vi "Read SCH Array Parameters.vi"(7 "FPGA Configuration Values In":T1={"Ln2 Filter Size"=10, "VT Quench Tick Limit"=4000000, "VT Quench Volt Limit"=0.1999969482421875, "Joint Tick Limit"=4000000, "Joint Volt Limit"=9.98377799987793e-07, "CoWound Volt Limit"=0.20001220703125, "CoWound Tick Limit"=4000000, "SC Bus Limit"=0.001953125, "SC Bus Tick Limit"=4000000, "ResMag Tick Limit"=1000000, "DAQ Cycle Ticks"=4096, "Res Mag dI/dt Delay"=256, "dI/dT scaling"=38.14697265625, "Pressure Inlet Limit (BarA)"=6.0, "Bore Tube Volt Limit"=0.5999999940395355, "Pressure Outlet Limit (BarA)"=5.0, "Activation Current (kA)"=0.5, "Dump Resistor Scale Factor"=200.0, "Co-Wound Asymmetry Factor"=0.0, "Co-Wound Scale Factor"=200.0, "Layer Scale Factors"=[3.0, 3.0, 3.0, 3.0, 3.0, 3.0, 3.0, 3.0, 3.0, 3.0, 3.0, 3.0, 3.0, 3.0, 3.0, 3.0, 3.0, 3.0], "Fudge Factors"=[0.0, 0.0, 0.0, 0.0, 0.0, 0.0, 0.0, 0.0, 0.0, 0.0, 0.0, 0.0, 0.0, 0.0, 0.0, 0.0], "Joint Scale Factors"=[1.0013580322265625e-05, 1.0013580322265625e-05, 1.0013580322265625e-05, 1.0013580322265625e-05, 1.0013580322265625e-05, 1.0013580322265625e-05, 1.0013580322265625e-05, 1.0013580322265625e-05], "SC Bus Scale"=[0.0009765326976776123, 0.0009765326976776123, 0.0009765326976776123, 0.0009765326976776123, 0.0009765326976776123, 0.0009765326976776123], "Pressure Scale Factor"=[1.723690003156662, 1.723690003156662, 1.723690003156662, 1.723690003156662], "# Consecutive Zeros Fault"=1000, "Digitize Convert Ticks"=200, "Digitize Reset Ticks"=400, "Convert Clock Ticks"=20, "Digitize Read Delay Ticks"=13, "Digitize # Bits"=16, "HTS Lead Tick Limit"=4000000, "Res Lead Tick Limit"=4000000, "HTS Lead Trip"=0.20000000298023224, "Res Lead Limit"=0.001953125, "HTS Lead FRZ"=0.006999999284744263, "HTS Lead Warn"=0.0010000020265579224} {"HTS Lead Warn" format="%_6g"; "HTS Lead FRZ" format="%_6g"; "Res Lead Limit" format="%_6g"; "HTS Lead Trip" format="%_6g"; "Pressure Scale Factor" format="%_6g"; "Fudge Factors" format="%.4g"; "Co-Wound Asymmetry Factor" format="%.8g"; "Activation Current (kA)" format="%_6g"; "Pressure Outlet Limit (BarA)" format="%.5g"; "Bore Tube Volt Limit" format="%_6g"; "Pressure Inlet Limit (BarA)" format="%.5g"; "dI/dT scaling" format="%.11g"; "SC Bus Limit" format="%_6g"; "Joint Volt Limit" format="%_6g"; "VT Quench Volt Limit" format="%.5g"}, 8 "error in (no error)":errorcluster, 9 "section":string, 10 "refnum in":T16) -> (0 "error out":errorcluster, 2 "refnum out":T16, 5 "FPGA Configuration Values Out":T1={"Ln2 Filter Size"=10, "VT Quench Tick Limit"=4000000, "VT Quench Volt Limit"=0.1999969482421875, "Joint Tick Limit"=4000000, "Joint Volt Limit"=9.98377799987793e-07, "CoWound Volt Limit"=0.20001220703125, "CoWound Tick Limit"=4000000, "SC Bus Limit"=0.001953125, "SC Bus Tick Limit"=4000000, "ResMag Tick Limit"=1000000, "DAQ Cycle Ticks"=4096, "Res Mag dI/dt Delay"=256, "dI/dT scaling"=38.14697265625, "Pressure Inlet Limit (BarA)"=6.0, "Bore Tube Volt Limit"=0.5999999940395355, "Pressure Outlet Limit (BarA)"=5.0, "Activation Current (kA)"=0.5, "Dump Resistor Scale Factor"=200.0, "Co-Wound Asymmetry Factor"=0.0, "Co-Wound Scale Factor"=200.0, "Layer Scale Factors"=[3.0, 3.0, 3.0, 3.0, 3.0, 3.0, 3.0, 3.0, 3.0, 3.0, 3.0, 3.0, 3.0, 3.0, 3.0, 3.0, 3.0, 3.0], "Fudge Factors"=[0.0, 0.0, 0.0, 0.0, 0.0, 0.0, 0.0, 0.0, 0.0, 0.0, 0.0, 0.0, 0.0, 0.0, 0.0, 0.0], "Joint Scale Factors"=[1.0013580322265625e-05, 1.0013580322265625e-05, 1.0013580322265625e-05, 1.0013580322265625e-05, 1.0013580322265625e-05, 1.0013580322265625e-05, 1.0013580322265625e-05, 1.0013580322265625e-05], "SC Bus Scale"=[0.0009765326976776123, 0.0009765326976776123, 0.0009765326976776123, 0.0009765326976776123, 0.0009765326976776123, 0.0009765326976776123], "Pressure Scale Factor"=[1.723690003156662, 1.723690003156662, 1.723690003156662, 1.723690003156662], "# Consecutive Zeros Fault"=1000, "Digitize Convert Ticks"=200, "Digitize Reset Ticks"=400, "Convert Clock Ticks"=20, "Digitize Read Delay Ticks"=13, "Digitize # Bits"=16, "HTS Lead Tick Limit"=4000000, "Res Lead Tick Limit"=4000000, "HTS Lead Trip"=0.20000000298023224, "Res Lead Limit"=0.001953125, "HTS Lead FRZ"=0.006999999284744263, "HTS Lead Warn"=0.0010000020265579224} {"HTS Lead Warn" format="%_6g"; "HTS Lead FRZ" format="%_6g"; "Res Lead Limit" format="%_6g"; "HTS Lead Trip" format="%_6g"; "Pressure Scale Factor" format="%_6g"; "Fudge Factors" format="%.4g"; "Co-Wound Asymmetry Factor" format="%.8g"; "Activation Current (kA)" format="%_6g"; "Pressure Outlet Limit (BarA)" format="%.5g"; "Bore Tube Volt Limit" format="%_6g"; "Pressure Inlet Limit (BarA)" format="%.5g"; "dI/dT scaling" format="%.11g"; "SC Bus Limit" format="%_6g"; "Joint Volt Limit" format="%_6g"; "VT Quench Volt Limit" format="%.5g"})   [LabVIEW 2017]
doc: "Author: Scott Hannahs <sth@magnet.fsu.edu>\nCopyright 2018 Florida State University, All rights reserved."
uses:
  <vilib>/Utility/config.llb/NI_LVConfig.lvlib
  <vilib>/Utility/config.llb/Read Key (String).vi
  <vilib>/Utility/config.llb/Config Data RefNum.ctl
  SCH Data Controls/SCH FXP Type.ctl
  SCH Data Controls/SCH Data 2 RT.ctl
  SCH Test Controls/SCH CoWound Volt Limit.ctl
  SCH Scaling Controls/SCH Dump Resistor Scale Factor.ctl
  SCH Test Controls/SCH CoWound Geometric Factor.ctl
  SCH Scaling Controls/SCH CoWound Scale Factor.ctl
  SCH Scaling Controls/SCH Scale Factor.ctl
  SCH Scaling Controls/SCH Scale Factor Array.ctl
  SCH Test Controls/SCH Fudge Factor.ctl
  SCH Test Controls/SCH Fudge Factor Array.ctl
  SCH Scaling Controls/SCH Joint Scale Factor.ctl
  SCH Scaling Controls/SCH Joint Scale Factor Array.ctl
  SCH Scaling Controls/SCH SC Bus Scale Factor.ctl
  SCH Scaling Controls/SCH SC Bus Scale Factor Array.ctl
  SCH Data Controls/FPGA Configure Parameters.ctl
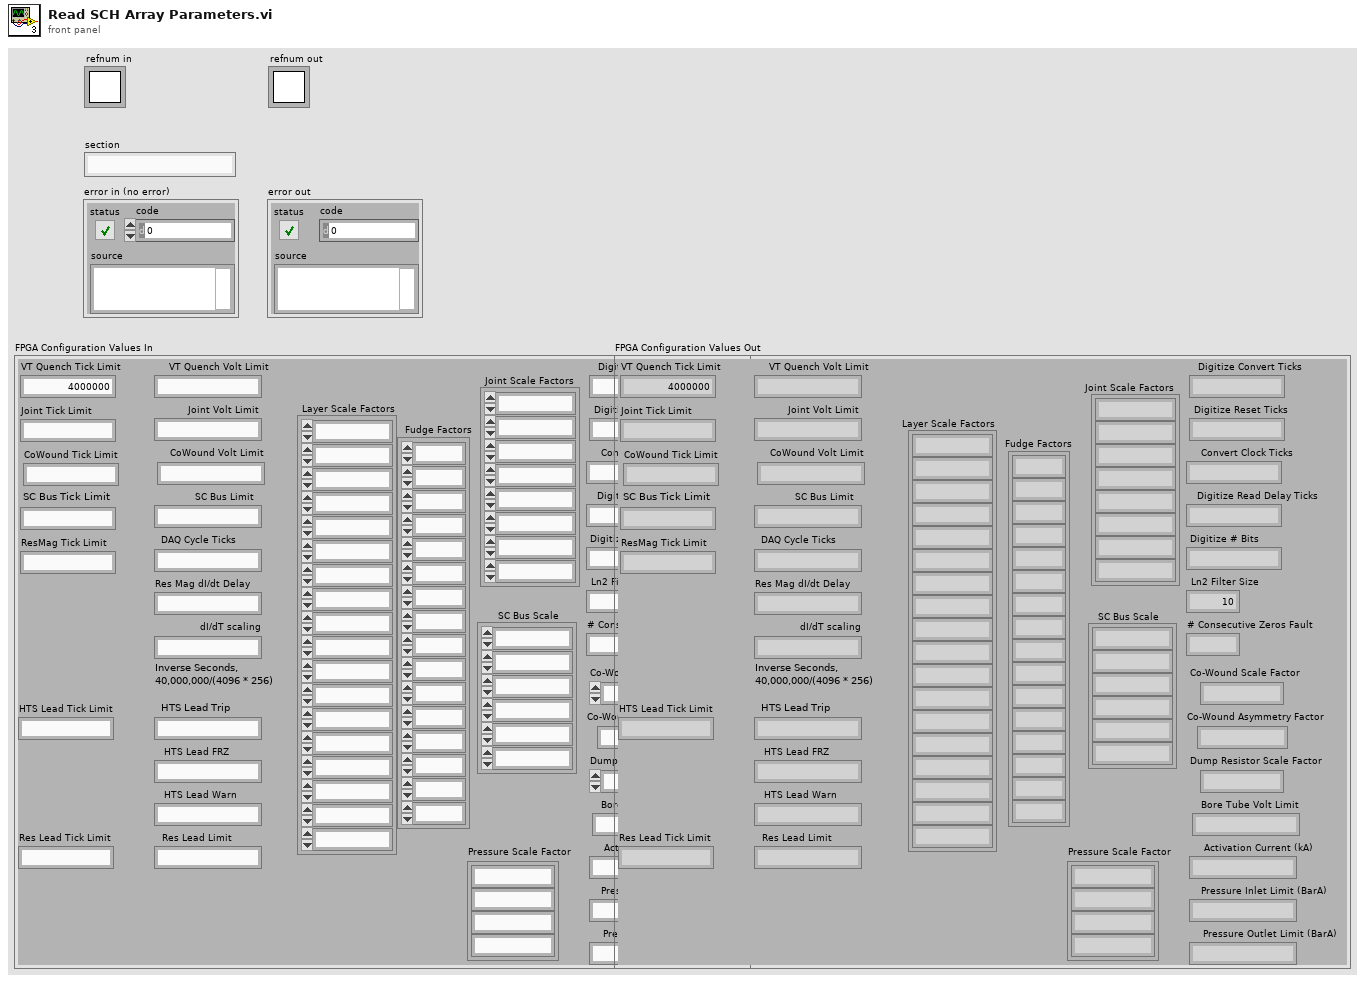
[diagram p1: front panel]
types:
  T1 = typedef "FPGA Configure Parameters.ctl" = cluster{"Ln2 Filter Size":i16, "VT Quench Tick Limit":u32, "VT Quench Volt Limit":T2, "Joint Tick Limit":u32, "Joint Volt Limit":T3, "CoWound Volt Limit":T4, "CoWound Tick Limit":u32, "SC Bus Limit":T3, "SC Bus Tick Limit":u32, "ResMag Tick Limit":u32, "DAQ Cycle Ticks":u32, "Res Mag dI/dt Delay":u32, "dI/dT scaling":fxp<+/-,35,11>, "Pressure Inlet Limit (BarA)":T2, "Bore Tube Volt Limit":T3, "Pressure Outlet Limit (BarA)":T2, "Activation Current (kA)":T3, "Dump Resistor Scale Factor":T5, "Co-Wound Asymmetry Factor":T6, "Co-Wound Scale Factor":T7, "Layer Scale Factors":T8, "Fudge Factors":T10, "Joint Scale Factors":T12, "SC Bus Scale":T14, "Pressure Scale Factor":T3[], "# Consecutive Zeros Fault":i16, "Digitize Convert Ticks":u32, "Digitize Reset Ticks":u32, "Convert Clock Ticks":u32, "Digitize Read Delay Ticks":u32, "Digitize # Bits":u32, "HTS Lead Tick Limit":u32, "Res Lead Tick Limit":u32, "HTS Lead Trip":T3, "Res Lead Limit":T3, "HTS Lead FRZ":T3, "HTS Lead Warn":T3}
  T2 = typedef "SCH FXP Type.ctl" = fxp<+/-,32,16>
  T3 = typedef "SCH Data 2 RT.ctl" = fxp<+/-,38,12>
  T4 = typedef "SCH CoWound Volt Limit.ctl" = fxp<+/-,16,1>
  T5 = typedef "SCH Dump Resistor Scale Factor.ctl" = fxp<+/-,38,12>
  T6 = typedef "SCH CoWound Geometric Factor.ctl" = fxp<+/-,16,0>
  T7 = typedef "SCH CoWound Scale Factor.ctl" = fxp<+/-,38,12>
  T8 = typedef "SCH Scale Factor Array.ctl" = T9[]
  T9 = typedef "SCH Scale Factor.ctl" = fxp<+/-,38,12>
  T10 = typedef "SCH Fudge Factor Array.ctl" = T11[]
  T11 = typedef "SCH Fudge Factor.ctl" = fxp<+/-,32,3>
  T12 = typedef "SCH Joint Scale Factor Array.ctl" = T13[]
  T13 = typedef "SCH Joint Scale Factor.ctl" = fxp<+/-,38,12>
  T14 = typedef "SCH SC Bus Scale Factor Array.ctl" = T15[]
  T15 = typedef "SCH SC Bus Scale Factor.ctl" = fxp<+/-,38,12>
  T16 = typedef "NI_LVConfig.lvlib/Config Data RefNum.ctl" = refnum<k1>
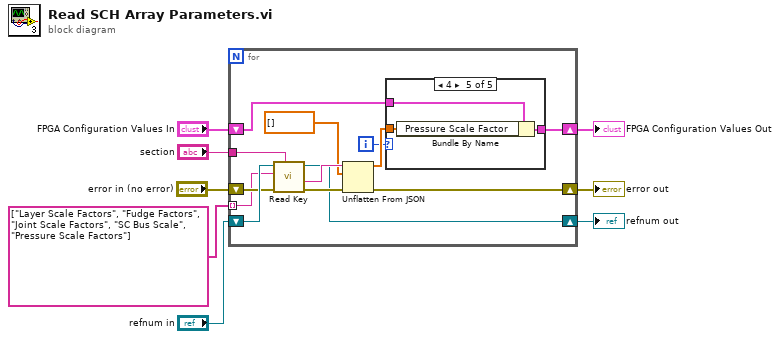
[diagram p0: block diagram]
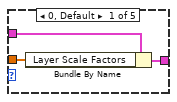
[diagram p2: hidden frame]
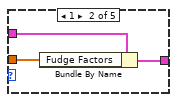
[diagram p3: hidden frame]
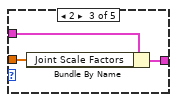
[diagram p4: hidden frame]
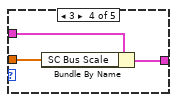
[diagram p5: hidden frame]
diagram:
  n1 = for {
    tunnel: "section" -> [w19]
    tunnel: string[] ["Layer Scale Factors", "Fudge Factors", "Joint Scale Factors", "SC Bus Scale", "Pressure Scale Factors"] ("key") -> [w15] mode=indexing
    shift-right: [w11] -> w7
    shift-left: "error in (no error)" -> [w20]
    shift-right: [w13] -> w8
    shift-left: "refnum in" -> [w21]
    shift-right: [w10] -> w2
    shift-left: "FPGA Configuration Values In" -> [w9]
    i -> [w12]
    n2 = call-poly <vilib>:"Read Key.vi"("section"=w19, "error in (no error)"=w20, "key"=w15, "refnum"=w21) -> ("error out"=w17:errorcluster, "value"=w18:string, "refnum out"=w13:T16)  [unwired: 4 in, 1 out]
    n3 = Unflatten From JSON(JSON string=w18, type and defaults=dbl[] [], error in (no error)=w17) -> (value=w14:dbl[], error out=w11:errorcluster)  [unwired: 4 in]
    n4 = case shown="4" w12 {
      tunnel: w14 -> [w22 w25 w28 w31 w34]
      tunnel: [w24 w27 w30 w33 w36] -> w10
      tunnel: w9 -> [w23 w26 w29 w32 w35]
      frame 0, Default {
        n5 = Bundle By Name(cluster=w23, "Layer Scale Factors"=w22) -> (w24:T1)
      }
      frame 1 {
        n6 = Bundle By Name(cluster=w26, "Fudge Factors"=w25) -> (w27:T1)
      }
      frame 2 {
        n7 = Bundle By Name(cluster=w29, "Joint Scale Factors"=w28) -> (w30:T1)
      }
      frame 3 {
        n8 = Bundle By Name(cluster=w32, "SC Bus Scale"=w31) -> (w33:T1)
      }
      frame 4 {
        n9 = Bundle By Name(cluster=w35, "Pressure Scale Factor"=w34) -> (w36:T1)
      }
    }
  }
  "refnum out" <- w8
  "error out" <- w7
  "FPGA Configuration Values Out" <- w2
